vi "Close.vi"(8 "error in (no error)":errorcluster, 11 "PLC in":refnum<class "MB PLC Client.lvclass">) -> (0 "error out":errorcluster, 3 "PLC out":refnum<class "MB PLC Client.lvclass">)   [LabVIEW 2018, in "MB PLC Client.lvlib" / "MB PLC Client.lvclass"]
uses:
  MB PLC Client.lvclass
  MB PLC Client.lvclass/MB PLC Client.ctl
  <vilib>/Plasmionique/MB Master/MB_Master/MB_Master.lvclass
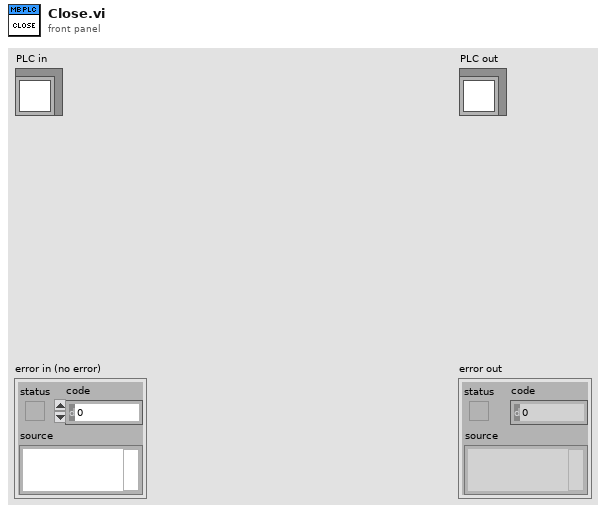
[diagram p1: front panel]
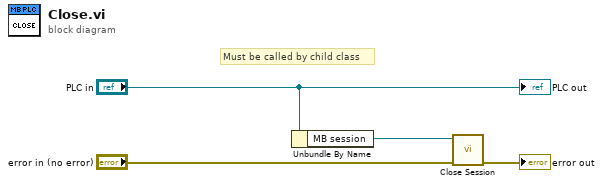
[diagram p0: block diagram]
diagram:
  # "Must be called by child class"
  n1 = Unbundle By Name("PLC in") -> ("MB session"=w3:refnum<class "MB_Master.lvclass">)
  n2 = call-dynamic "Close Session.vi"("error in (no error)"="error in (no error)", "MB session in"=w3) -> ("error out"=→"error out":errorcluster)  [unwired: 9 in]
  "PLC out" <- "PLC in"
